vi "自动升级更新main.vi"() -> ()   [LabVIEW 2016, in "数据传输系统.lvlib"]
panel:
  out "waittime":u8
  out "有新版本":bool
  out "下载的文件名":string
  out "最新版本获取进度":u8(slide) scale=0.0..100.0
  # "版本获取中，请稍后！"
  # "s"
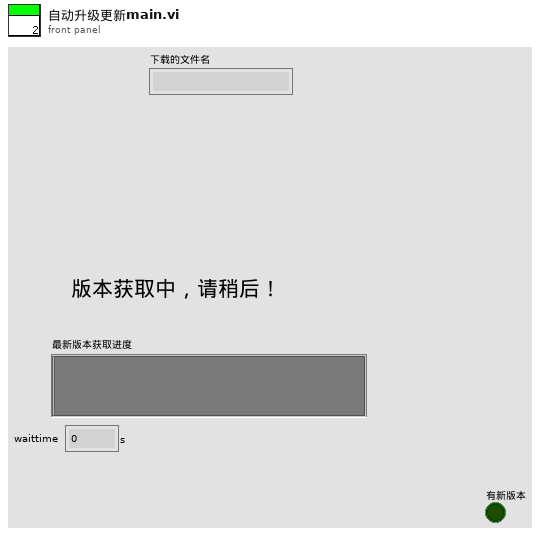
[diagram p1: front panel]
types:
  T1 = enum16{"get version information", "get success", "contact", "over"}
  T2 = enum16{"open", "replace", "create", "open or create", "replace or create", "replace or create with confirmation"}
  T3 = cluster{"网络灯":bool, "接收中":bool, "已接收百分比":u8, "接收成功次数":dbl, "当前步骤":enum16{"init", "receivehead", "receivecontent", "receivesuccess", "over"}, "文件名":string, "error out":errorcluster}
  T4 = enum32{"Bad", "Idle", "Run top level", "Running"}
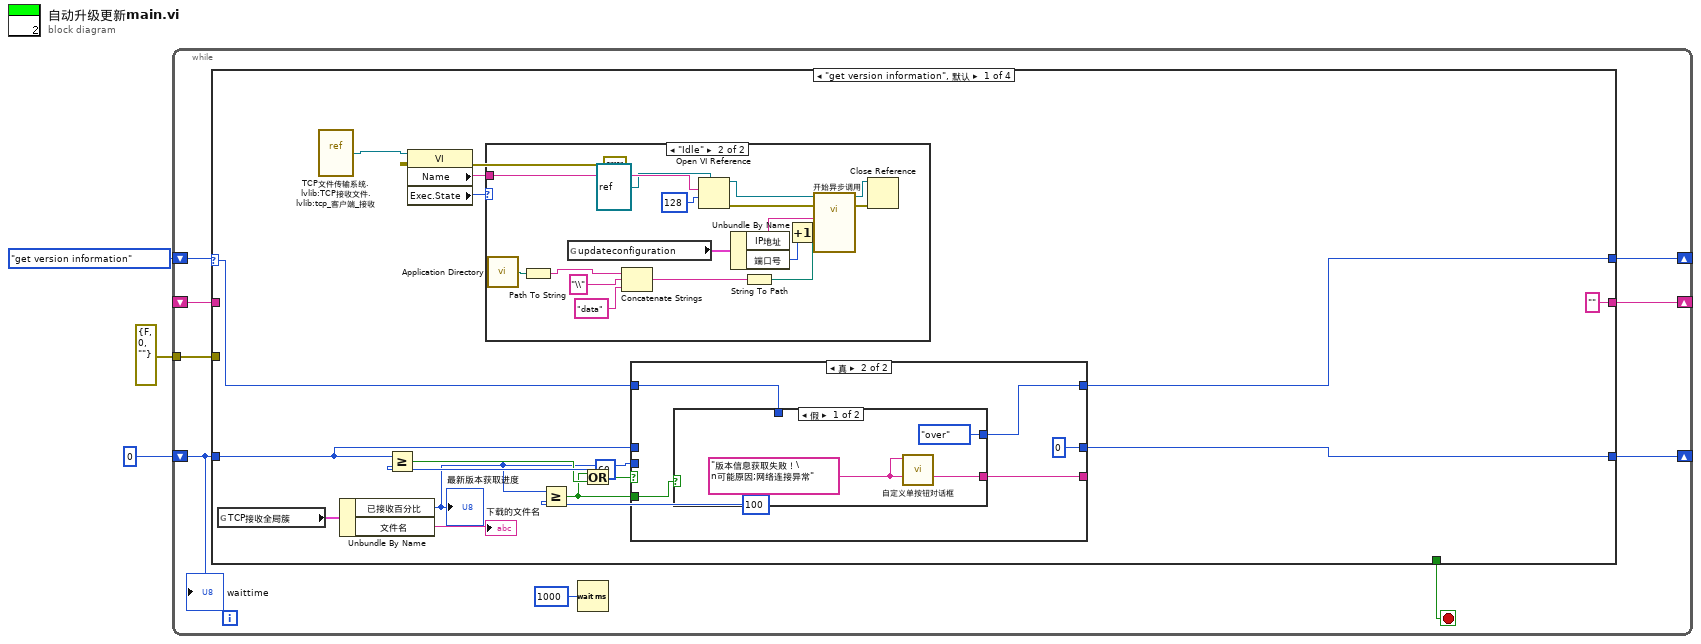
[diagram p0: block diagram]
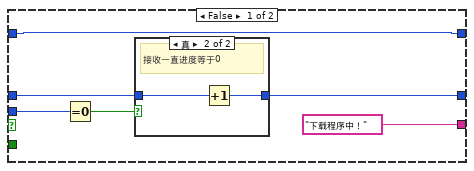
[diagram p2: hidden frame]
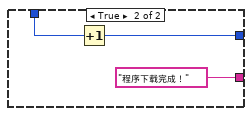
[diagram p4: hidden frame]
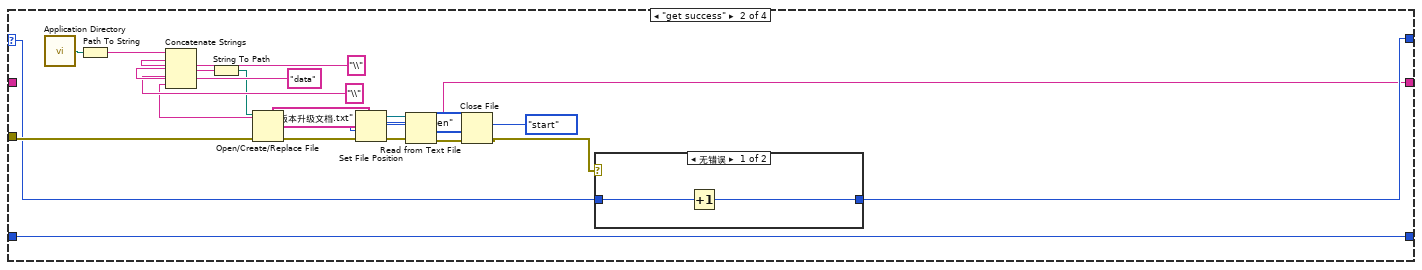
[diagram p6: hidden frame]
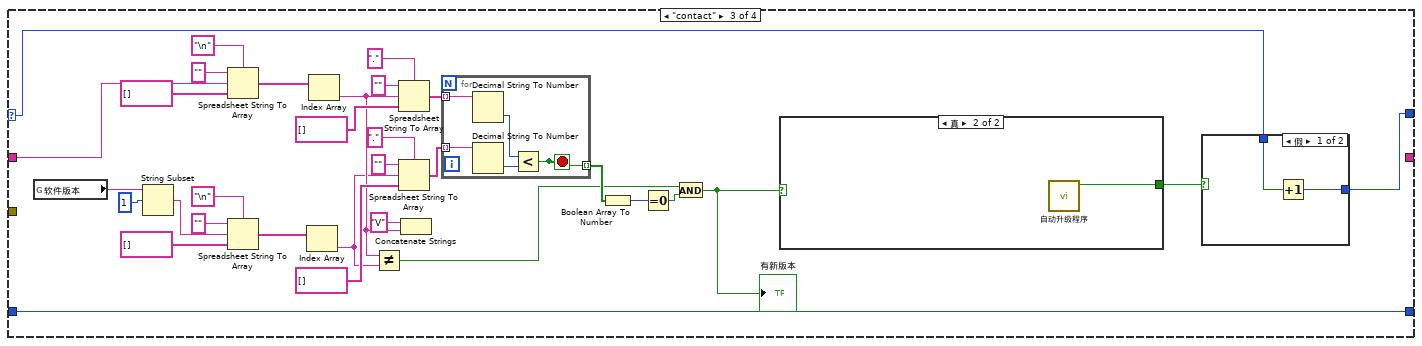
[diagram p8: hidden frame]
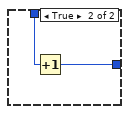
[diagram p9: hidden frame]
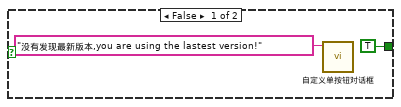
[diagram p10: hidden frame]
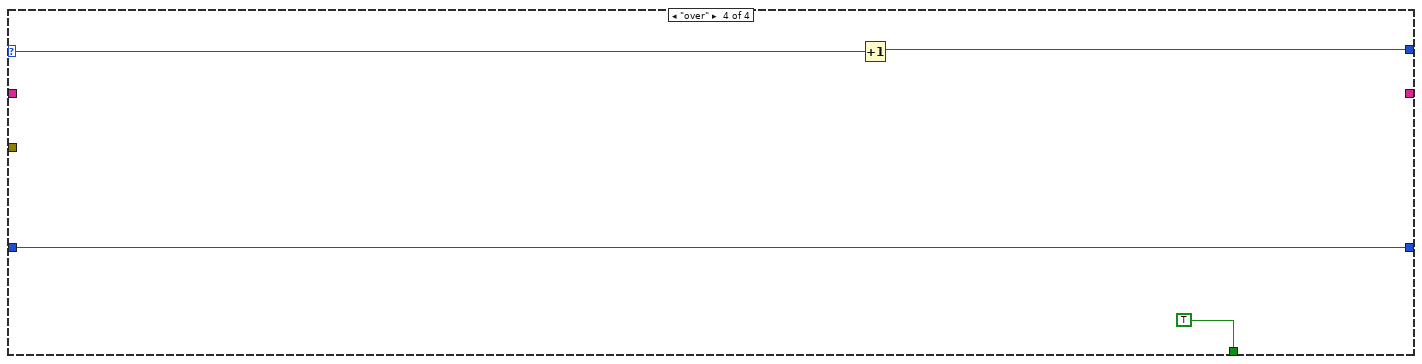
[diagram p11: hidden frame]
diagram:
  n1 = while {
    shift-right: [w8] -> _
    shift-left: T1."get version information" -> [w11]
    shift-right: [w9] -> _
    shift-left: u8 0 ("y") -> [w10]
    tunnel: errorcluster {"status"=FALSE, "code"=0, "source"=""} ("错误常量") -> [w7]
    shift-right: [w6] -> _
    shift-left: _ -> [w5]
    stop <- w4 stop-if-true
    n2 = case shown="\"get version information\", 默认" w11 {
      selector: w11 -> [w15 w74 w93 w136]
      tunnel: w10 -> [w17 w66 w91 w137]
      tunnel: [w16 w66 w91 w137] -> w9
      tunnel: [w14 w73 w92 w135] -> w8
      tunnel: w7 -> [_ w75 _ _]
      tunnel: ["" w67 _ _] -> w6
      tunnel: w5 -> [_ _ w96 _]
      tunnel: [_ _ _ TRUE] -> w4
      frame "get version information", Default {
        n3 = global read "全局变量1.vi" "TCP接收全局簇"() -> (w20:T3)
        n4 = vi-ref "TCP文件传输系统.lvlib:TCP接收文件.lvlib:tcp_客户端_接收.vi"() -> (w29:refnum<vi>)
        n5 = Unbundle By Name(w20) -> ("已接收百分比"=w21:u8, "文件名"=→"下载的文件名":string)
        "最新版本获取进度" <- w21
        n6 = Greater Or Equal?(x=w17, y=u8 60) -> (x >= y?=w23:bool)
        n7 = property class="VI"(reference=w29, error in=errorcluster {"status"=FALSE, "code"=0, "source"=""} ("错误输出")) -> ("Name"=w28:string, "Exec.State"=w26:T4)  [unwired: 2 out]
        n8 = case shown="\"Idle\"" w26 {
          tunnel: w28 -> [_ w65]
          frame "Bad", Default {
          }
          frame "Idle" {
            n9 = call <vilib>:"Application Directory.vi"() -> ("Application Directory"=w54:path)
            n10 = Path To String(path=w54) -> (string=w51:string)
            n11 = global read "update全局.vi" "updateconfiguration"() -> (w58:cluster{"IP地址":string, "端口号":i32})
            n12 = Concatenate Strings(w51, "\\" ("字符串"), "data" ("字符串")) -> (w55:string)
            n13 = Open VI Reference(type specifier VI Refnum (for type only)=refnum<vi> refnum, vi path=w65, options=128 ("选项")) -> (vi reference=w63:refnum<vi>, error out=w61:errorcluster)  [unwired: 3 in]
            n14 = Unbundle By Name(w58) -> ("IP地址"=w57:string, "端口号"=w56:i32)
            n15 = String To Path(string=w55) -> (path=w50:path)
            n16 = Increment(x=w56) -> (x+1=w49:i32)
            n17 = call-by-ref "开始异步调用"(reference=w63, error in=w61, "IP地址"=w57, "端口号"=w49, "储存路径"=w50) -> (reference out=w59:refnum<vi>, error out=w60:errorcluster)  [unwired: 17 in]
            n18 = Close Reference(reference=w59, error in (no error)=w60) -> ()  [unwired: 1 out]
          }
        }
        n19 = Greater Or Equal?(x=w21, y=u8 100) -> (x >= y?=w19:bool)
        n20 = Or(x=w19, y=w23) -> (x .or. y?=w22:bool)
        n21 = case shown="真" w22 {
          tunnel: w17 -> [w35 _]
          tunnel: [w34 u8 0] -> w16
          tunnel: w21 -> [w32 _]
          tunnel: [w31 w39] -> w14
          tunnel: w15 -> [w31 w40]
          tunnel: ["下载程序中！" w41] -> _
          tunnel: w19 -> [_ w42]
          frame False {
            n22 = Equal To 0?(x=w32) -> (x = 0?=w33:bool)
            n23 = case shown="真" w33 {
              tunnel: w35 -> [w36 w38]
              tunnel: [w36 w37] -> w34
              frame False {
              }
              frame True {
                # "接收一直进度等于0"
                n24 = Increment(x=w38) -> (x+1=w37:u8)
              }
            }
          }
          frame True {
            n25 = case shown="假" w42 {
              tunnel: [w45 "程序下载完成！"] -> w41
              tunnel: w40 -> [_ w47]
              tunnel: [T1."over" w46] -> w39
              frame False {
                w45 = "版本信息获取失败！\n可能原因;网络连接异常"
                n26 = call "自定义单按钮对话框.vi"("消息"=w45) -> ()  [unwired: 11 in]
              }
              frame True {
                n27 = Increment(x=w47) -> (x+1=w46:T1)
              }
            }
          }
        }
      }
      frame "get success" {
        n28 = call <vilib>:"Application Directory.vi"() -> ("Application Directory"=w80:path)
        n29 = Path To String(path=w80) -> (string=w83:string)
        n30 = Concatenate Strings(w83, "\\" ("字符串"), "data" ("字符串"), "\\" ("字符串"), "版本升级文档.txt" ("字符串")) -> (w77:string)
        n31 = String To Path(string=w77) -> (path=w76:path)
        n32 = Open/Create/Replace File(file path (use dialog)=w76, error in=w75, operation (0:open)=T2."open" ("操作(0:open)")) -> (refnum out=w86:refnum<file>, error out=w85:errorcluster)  [unwired: 3 in, 1 out]
        n33 = Set File Position(refnum=w86, from (0:start)=enum16{"start", "end", "current"}."start" ("自（0:起始）"), error in=w85) -> (refnum out=w71:refnum<file>, error out=w70:errorcluster)  [unwired: 1 in]
        n34 = Read from Text File(file (use dialog)=w71, error in=w70) -> (refnum out=w72:refnum<file>, text=w67:string, error out=w69:errorcluster)  [unwired: 2 in, 1 out]
        n35 = Close File(refnum=w72, error in=w69) -> (error out=w68:errorcluster)  [unwired: 1 out]
        n36 = case shown="无错误" w68 {
          tunnel: w74 -> [w89 w90]
          tunnel: [w88 w90] -> w73
          frame No Error {
            n37 = Increment(x=w89) -> (x+1=w88:T1)
          }
          frame Error {
          }
        }
      }
      frame "contact" {
        n38 = global read "update全局.vi" "软件版本"() -> (w114:string)
        n39 = String Subset(string=w114, offset (0)=1 ("偏移量(0)")) -> (substring=w109:string)  [unwired: 1 in]
        n40 = Spreadsheet String To Array(delimiter (Tab)="\n" ("分隔符(Tab)"), format string="" ("格式字符串"), spreadsheet string=w96, array type (2D Dbl)=string[] []) -> (array=w118:string[])
        n41 = Spreadsheet String To Array(delimiter (Tab)="\n" ("分隔符(Tab)"), format string="" ("格式字符串"), spreadsheet string=w109, array type (2D Dbl)=string[] []) -> (array=w108:string[])
        n42 = Index Array(array=w108) -> (element=w99:string)  [unwired: 1 in]
        n43 = Index Array(array=w118) -> (element=w100:string)  [unwired: 1 in]
        n44 = Not Equal?(x=w100, y=w99) -> (x != y?=w97:bool)
        n45 = Spreadsheet String To Array(delimiter (Tab)="." ("分隔符(Tab)"), format string="" ("格式字符串"), spreadsheet string=w100, array type (2D Dbl)=string[] []) -> (array=w104:string[])
        n46 = Spreadsheet String To Array(delimiter (Tab)="." ("分隔符(Tab)"), format string="" ("格式字符串"), spreadsheet string=w99, array type (2D Dbl)=string[] []) -> (array=w103:string[])
        n47 = Concatenate Strings("V" ("字符串"), w100) -> ()  [unwired: 1 out]
        n48 = for {
          tunnel: w104 -> [w132] mode=indexing
          tunnel: w103 -> [w134] mode=indexing
          tunnel: [w133] -> w102 mode=indexing
          stop <- w133 stop-if-true
          n49 = Decimal String To Number(string=w132) -> (number=w131:i32)  [unwired: 2 in, 1 out]
          n50 = Decimal String To Number(string=w134) -> (number=w130:i32)  [unwired: 2 in, 1 out]
          n51 = Less?(x=w131, y=w130) -> (x < y?=w133:bool)
        }
        n52 = Boolean Array To Number(Boolean array=w102) -> (number=w101:u32)
        n53 = Equal To 0?(x=w101) -> (x = 0?=w98:bool)
        n54 = And(x=w97, y=w98) -> (x .and. y?=w95:bool)
        "有新版本" <- w95
        n55 = case shown="真" w95 {
          tunnel: [TRUE ("确定") w129] -> w94
          frame False {
            n56 = call "自定义单按钮对话框.vi"("消息"="没有发现最新版本,you are using the lastest version!") -> ()  [unwired: 11 in]
          }
          frame True {
            n57 = call "自动升级程序.vi"() -> ("确定"=w129:bool)  [unwired: 10 in, 1 out]
          }
        }
        n58 = case shown="假" w94 {
          tunnel: w93 -> [w124 w126]
          tunnel: [w123 w125] -> w92
          frame False {
            n59 = Increment(x=w124) -> (x+1=w123:T1)
          }
          frame True {
            n60 = Increment(x=w126) -> (x+1=w125:T1)
          }
        }
      }
      frame "over" {
        n61 = Increment(x=w136) -> (x+1=w135:T1)
      }
    }
    n62 = Wait (ms)(milliseconds to wait=u32 1000 ("等待时间（毫秒）")) -> ()  [unwired: 1 out]
    "waittime" <- w10
  }
